vi "XLP80_Action_WriteChannelRings.vi"() -> ()   [LabVIEW 2021]
uses:
  XLP80_FGlob/XLP80_FGlob_TDefEnumCANReadItems.ctl
  XLP80_FGlob/XLP80_FGlob_TDefEnumcDAQDOItems.ctl
  XLP80_FGlob/XLP80_FGlob_TDefEnumcDAQDIItems.ctl
  XLP80_FGlob/XLP80_FGlob_TDefEnumcDAQAIItems.ctl
panel:
  in  "cDAQ AI Item":T1
  in  "cDAQ DI Item":T2
  in  "cDAQ DO Item":T3
  in  "Tab Control":enum32{"DI", "DO", "AI", "TC", "AO", "CAN"}(tab)
  in  "cDAQ DI Item":u16(ring) items=["Heizeinheit_Stoerung", "E-Erhitzer_Betrieb", "Dosierpumpe_Betrieb", "5_2_Wegeventil_hoch_Rueckmeldung", "5_2_Wegeventil_runter_Rueckmeldung", "Not-Aus", "Reserve_DI_4_6", "Reserve_DI_4_7"]
  in  "Signal Name":string[](array[string])=["EK_TS", "EZ_Um1", "EZ_Um2", "EZ_Um3", "WZ_TS", "NP", "LP", "HP", "ROP", "CO2P", "WP", "EZ_IW", "ESTB_LB", "ESTB_HB", "ESTB_WB", "ESTB_H1", "WZ_Pu", "KWZ_St", "KL_LAB", "KL_HAB", "KWLo_WB", "KWLu_WB", "WLo_LB", "WLu_LB", "WLo_HB", "WLu_HB", "EZ_TK1-3", "Res_5", "Res_4", "Res_3", "Res_2", "Res_1"]
  in  "Signal Name":string[](array[string])
  in  "cDAQ DO Item":u16(ring) items=["E-Erhitzer_Freigabe", "Reserve_DO_5_1", "5_2_Wegeventil_hoch_Freigabe", "5_2_Wegeventil_runter_Freigabe", "Dosierpumpe_EIN", "Reserve_DO_5_5", "Reserve_DO_5_6", "Reserve_DO_5_7"]
  in  "Signal Name":string[](array[string])=["AI0", "AI1", "AI2", "AI3"]
  in  "cDAQ AI Item":u16(ring) items=["Temperaturfuehler_01", "Temperaturfuehler_02", "Temperaturfuehler_03", "Temp_Ueberwachung_LEH", "Temp_LEH", "Reserve_TC_2_5", "Reserve_TC_2_6", "Reserve_TC_2_7", "Reserve_TC_2_8", "Reserve_TC_2_9", "Reserve_TC_2_10", "Reserve_TC_2_11", "Reserve_TC_2_12", "Reserve_TC_2_13", "Reserve_TC_2_14", "Reserve_TC_2_15", "Gasdosierung_1_Istwert", "Gasdosierung_2_Istwert", "Reserve_AI_2_2", "Reserve_AI_2_3", "Reserve_AI_2_4", "Reserve_AI_2_5", "Reserve_AI_2_6", "Reserve_AI_2_7"]
  in  "Signal Name":string[](array[string])
  in  "PXI TC Item":u16(ring)
  in  "Signal Name":string[](array[string])=["AO0", "AO1", "AO2", "AO3"]
  in  "cDAQ AO Item":u16(ring) items=["Drehzahl_Luefter", "Heizleistung_E-Erhitzer", "Gasdosierung_1_Sollwert", "Gasdosierung_2_Sollwert", "Reserve_AO_3_4", "Reserve_AO_3_5", "Reserve_AO_3_6", "Reserve_AO_3_7", "Reserve_AO_3_8", "Reserve_AO_3_9", "Reserve_AO_3_10", "Reserve_AO_3_11", "Reserve_AO_3_12", "Reserve_AO_3_13", "Reserve_AO_3_14", "Reserve_AO_3_15"]
  in  "CAN Read Items":T4
  in  "CAN Read Items":u16(ring) items=["F_P_H_SI", "F_T_S_0"]
  in  "Signal Name":string[](array[string])=["F_P_H_SI", "F_T_S_0"]
  # "Enum"
  # "Ring"
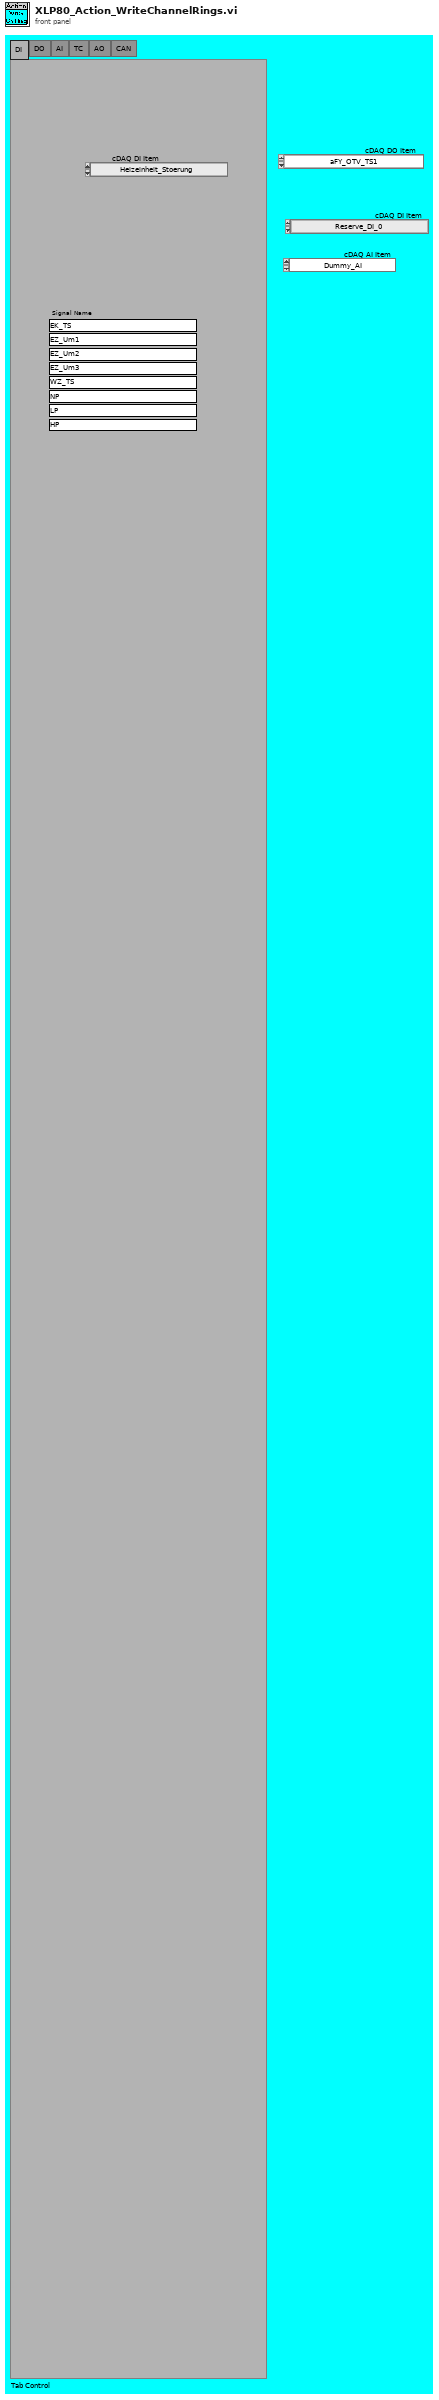
[diagram p1: front panel]
types:
  T1 = typedef "XLP80_FGlob_TDefEnumcDAQAIItems.ctl" = enum16{"Dummy_AI"}
  T2 = typedef "XLP80_FGlob_TDefEnumcDAQDIItems.ctl" = enum16{"Reserve_DI_0", "Reserve_DI_1", "Reserve_DI_2", "HcH_TS_Warn", "HcH_TS_Alarm", "Reserve_DI_5", "Reserve_DI_6", "Reserve_DI_7"}
  T3 = typedef "XLP80_FGlob_TDefEnumcDAQDOItems.ctl" = enum16{"aFY_OTV_TS1", "aEK_SRC_TS", "aFY_OTV_TS2", "Reserve_DO_3", "Reserve_DO_4", "Reserve_DO_5", "Reserve_DO_6", "Reserve_DO_7"}
  T4 = typedef "XLP80_FGlob_TDefEnumCANReadItems.ctl" = enum16{"F_P_H_SI_0", "F_T_S_0_0", "F_T_S_opt_0", "F_I_S_0", "F_CH_A_VO_0", "State_F_R_S_In_0", "State_F_SV_H_Si_0", "State_F_SV_H_So_0", "Purge_Time_0", "F_SV_H_SI_0", "F_R_S_0", "F_SV_H_So_0", "F_GP_A1_0", "F_GP_A2_0", "F_U_S_0", "F_RPM_V_0", "State_Set_EA_L0_0", "State_EA_L0_0", "State_EA_L1_0", "F_P_H_SI_1", "F_T_S_0_1", "F_T_S_opt_1", "F_I_S_1", "F_CH_A_VO_1", "State_F_R_S_In_1", "State_F_SV_H_Si_1", "State_F_SV_H_So_1", "Purge_Time_1", "F_SV_H_SI_1", "F_R_S_1", "F_SV_H_So_1", "F_GP_A1_1", "F_GP_A2_1", "F_U_S_1", "F_RPM_V_1", "State_Set_EA_L0_1", "State_EA_L0_1", "State_EA_L1_1", "F_P_H_SI_2", "F_T_S_0_2", "F_T_S_opt_2", "F_I_S_2", "F_CH_A_VO_2", "State_F_R_S_In_2", "State_F_SV_H_Si_2", "State_F_SV_H_So_2", "Purge_Time_2", "F_SV_H_SI_2", "F_R_S_2", "F_SV_H_So_2", "F_GP_A1_2", "F_GP_A2_2", "F_U_S_2", "F_RPM_V_2", "State_Set_EA_L0_2", "State_EA_L0_2", "State_EA_L1_2", "F_P_H_SI_3", "F_T_S_0_3", "F_T_S_opt_3", "F_I_S_3", "F_CH_A_VO_3", "State_F_R_S_In_3", "State_F_SV_H_Si_3", "State_F_SV_H_So_3", "Purge_Time_3", "F_SV_H_SI_3", "F_R_S_3", "F_SV_H_So_3", "F_GP_A1_3", "F_GP_A2_3", "F_U_S_3", "F_RPM_V_3", "State_Set_EA_L0_3", "State_EA_L0_3", "State_EA_L1_3", "F_P_H_SI_4", "F_T_S_0_4", "F_T_S_opt_4", "F_I_S_4", "F_CH_A_VO_4", "State_F_R_S_In_4", "State_F_SV_H_Si_4", "State_F_SV_H_So_4", "Purge_Time_4", "F_SV_H_SI_4", "F_R_S_4", "F_SV_H_So_4", "F_GP_A1_4", "F_GP_A2_4", "F_U_S_4", "F_RPM_V_4", "State_Set_EA_L0_4", "State_EA_L0_4", "State_EA_L1_4", "F_P_H_SI_5", "F_T_S_0_5", "F_T_S_opt_5", "F_I_S_5", "F_CH_A_VO_5", "State_F_R_S_In_5", "State_F_SV_H_Si_5", "State_F_SV_H_So_5", "Purge_Time_5", "F_SV_H_SI_5", "F_R_S_5", "F_SV_H_So_5", "F_GP_A1_5", "F_GP_A2_5", "F_U_S_5", "F_RPM_V_5", "State_Set_EA_L0_5", "State_EA_L0_5", "State_EA_L1_5", "F_P_H_SI_6", "F_T_S_0_6", "F_T_S_opt_6", "F_I_S_6", "F_CH_A_VO_6", "State_F_R_S_In_6", "State_F_SV_H_Si_6", "State_F_SV_H_So_6", "Purge_Time_6", "F_SV_H_SI_6", "F_R_S_6", "F_SV_H_So_6", "F_GP_A1_6", "F_GP_A2_6", "F_U_S_6", "F_RPM_V_6", "State_Set_EA_L0_6", "State_EA_L0_6", "State_EA_L1_6", "C_P_R_CAN_0", "C_U_E_CAN_0", "Initalisierung", "Stand_By", "Rack_Start", "Rack_In_Betrieb", "Rack_Shut_Down", "System_WARN", "System_EPO", "C_SV_H_T", "C_R_L", "C_R_R", "C_I_L_Set", "C_SV_H_R", "C_RPM_V_R", "C_T_A_R", "C_I_L", "C_p_H_Ri", "C_p_H_Ro", "C_p_H_T"}
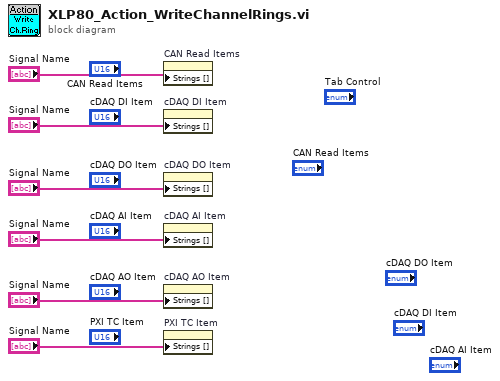
[diagram p0: block diagram]
diagram:
  n1 = property on="CAN Read Items" class="Ring (strict)"("Strings []"="Signal Name") -> ()  [unwired: 2 in, 2 out]
  n2 = property on="cDAQ DI Item" class="Ring (strict)"("Strings []"="Signal Name") -> ()  [unwired: 2 in, 2 out]
  n3 = property on="cDAQ DO Item" class="Ring (strict)"("Strings []"="Signal Name") -> ()  [unwired: 2 in, 2 out]
  n4 = property on="cDAQ AI Item" class="Ring (strict)"("Strings []"="Signal Name") -> ()  [unwired: 2 in, 2 out]
  n5 = property on="cDAQ AO Item" class="Ring (strict)"("Strings []"="Signal Name") -> ()  [unwired: 2 in, 2 out]
  n6 = property on="PXI TC Item" class="Ring (strict)"("Strings []"="Signal Name") -> ()  [unwired: 2 in, 2 out]
